vi "Nodos_propiedades_2.vi"() -> ()   [LabVIEW 2020]
panel:
  in  "stop":bool
  out "String":string
  out "Número de muestreos":i64
  in  "Límite de muestreo":i64
  in  "Límite superior":dbl
  in  "Tiempo de muestreo":dbl
  out "Fuera de rango":bool
  out "Temperatura":cluster{dbl, "Límite superior":dbl}(graph)
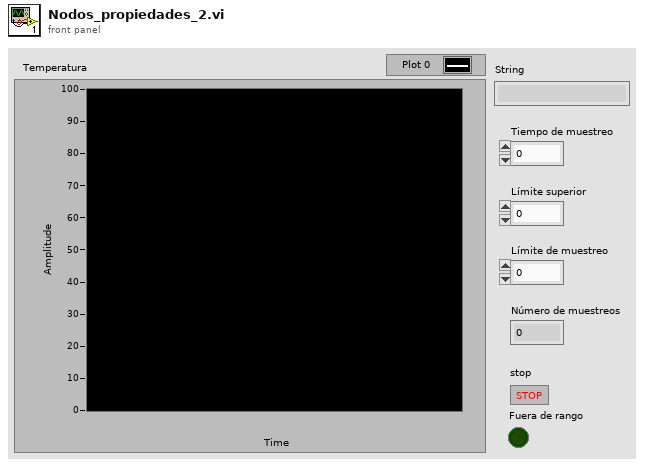
[diagram p1: front panel]
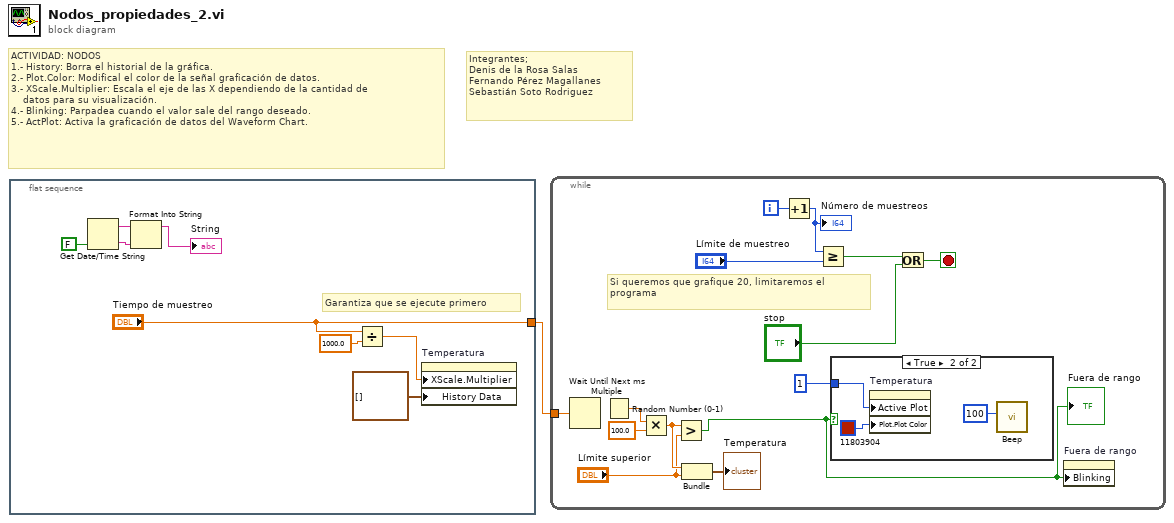
[diagram p0: block diagram]
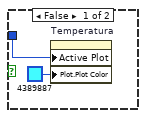
[diagram p2: hidden frame]
diagram:
  # "Integrantes;\nDenis de la Rosa Salas\nFernando Pérez Magallanes\nSebastián Soto Rodriguez"
  # "ACTIVIDAD: NODOS\n1.- History: Borra el historial de la gráfica.\n2.- Plot.Color: Modifical el color de la señal graficación de datos.\n3.- XScale.Multiplier: Escala el eje de las X dependiendo de la cantidad de\n    datos para su visualización.\n4.- Blinking: Parpadea cuando el valor sale del rango deseado.\n5.- ActPlot: Activa la graficación de datos del Waveform Chart."
  n1 = flat-sequence {
    tunnel: ["Tiempo de muestreo"] -> w1
    frame #0 {
      # "Garantiza que se ejecute primero"
      n2 = Get Date/Time String(want seconds? (F)=FALSE) -> (date string=w6:string, time string=w7:string)  [unwired: 2 in]
      n3 = Format Into String(initial string=w6, w7) -> (resulting string=→"String":string)  [unwired: 2 in, 1 out]
      n4 = Divide(x="Tiempo de muestreo", y=1000.0) -> (x/y=w5:dbl)
      n5 = property on="Temperatura" class="WFChart (strict)"("XScale.Multiplier"=w5, "History Data"=cluster{dbl, "Límite superior":dbl}[] []) -> ()  [unwired: 2 in, 2 out]
    }
  }
  n6 = while {
    tunnel: w1 -> [w23]
    i -> [w17]
    stop <- w15 stop-if-true
    # "Si queremos que grafique 20, limitaremos el\nprograma"
    n7 = Wait Until Next ms Multiple(millisecond multiple=w23) -> ()  [unwired: 1 out]
    n8 = Random Number (0-1)() -> (number: 0 to 1=w22:dbl)
    n9 = Multiply(x=w22, y=100.0) -> (x*y=w20:dbl)
    n10 = Greater?(x=w20, y="Límite superior") -> (0:w11:bool)
    "Fuera de rango" <- w11
    n11 = Bundle(w20, "Límite superior"="Límite superior") -> (→"Temperatura":cluster{dbl, "Límite superior":dbl})  [unwired: 1 in]
    n12 = Increment(x=w17) -> (x+1=w14:i32)
    "Número de muestreos" <- w14
    n13 = Greater Or Equal?(x=w14, y="Límite de muestreo") -> (x >= y?=w16:bool)
    n14 = case shown="True" w11 {
      tunnel: 1 -> [w25 w28]
      frame False {
        n15 = property on="Temperatura" class="WFChart (strict)"("Active Plot"=w25, "Plot.Plot Color"=u32 4389887) -> ()  [unwired: 2 in, 2 out]
      }
      frame True {
        n16 = property on="Temperatura" class="WFChart (strict)"("Active Plot"=w28, "Plot.Plot Color"=u32 11803904) -> ()  [unwired: 2 in, 2 out]
        n17 = call <vilib>:"Beep.vi"("duration (msec)"=u32 100) -> ()  [unwired: 11 in]
      }
    }
    n18 = Or(x=w16, y="stop") -> (x .or. y?=w15:bool)
    n19 = property on="Fuera de rango" class="Bool (strict)"("Blinking"=w11) -> ()  [unwired: 2 in, 2 out]
  }
